vi "Edit.TestLauncher.vi"() -> ()   [LabVIEW 2019, in "Edit.lvclass"]
uses:
  Edit.lvclass
  <vilib>/JKI/JKI SMO/SMO/Typedefs/SMOState --Enum.ctl
  C:/Program Files (x86)/National Instruments/LabVIEW 2019/vi.lib/JKI/JKI SMO/SMO/SMO.lvclass
  <vilib>/JKI/JKI SMO/SMO/SMO.lvclass/SMO.ctl
  <vilib>/JKI/JKI SMO/SMO/Private/ReftoDVR--SMO.vi
  <vilib>/JKI/JKI SMO/SMO/SMO.lvclass
panel:
  out "SMO State":T1
  out "error out":errorcluster
  in  "Stop":bool
  # "Basic SMO Test Launcher"
  # "For instructions on how to use the JKI State Machine Objects, examples and video tutorials, visit:\nhttp://jki.net/state-machine-objects/\n\nJKI State Machine Objects™\nhttp://jki.net/state-machine-objects/\nCopyright (C) 2005-2015, JKI <info@jki.net>\nALL RIGHTS RESERVED"
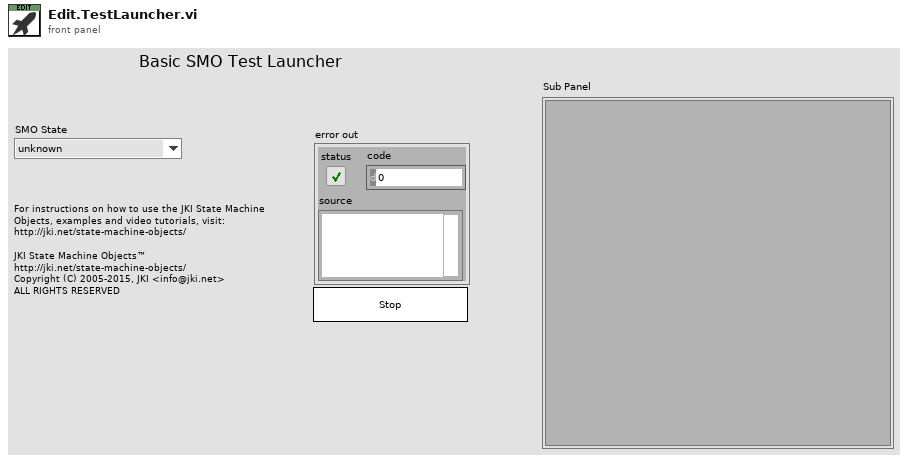
[diagram p1: front panel]
types:
  T1 = typedef "SMO.lvclass/SMOState --Enum.ctl" = enum16{"unknown", "Created", "Started", "Stopped"}
  T2 = typedef "SMO.lvclass/Public Events.ctl" = cluster{"Error":refnum<user-event>, "State":refnum<user-event>, "Reserve State":refnum<user-event>}
  T3 = cluster{"Event Registration Refnum":refnum<event-registration>}
  T4 = typedef "SMO.lvclass/RegisteredProcessData--Cluster.ctl" = cluster{"Name":string, "Static VI Ref":refnum<vi>, "Running":bool, "NotifierRef":u32}
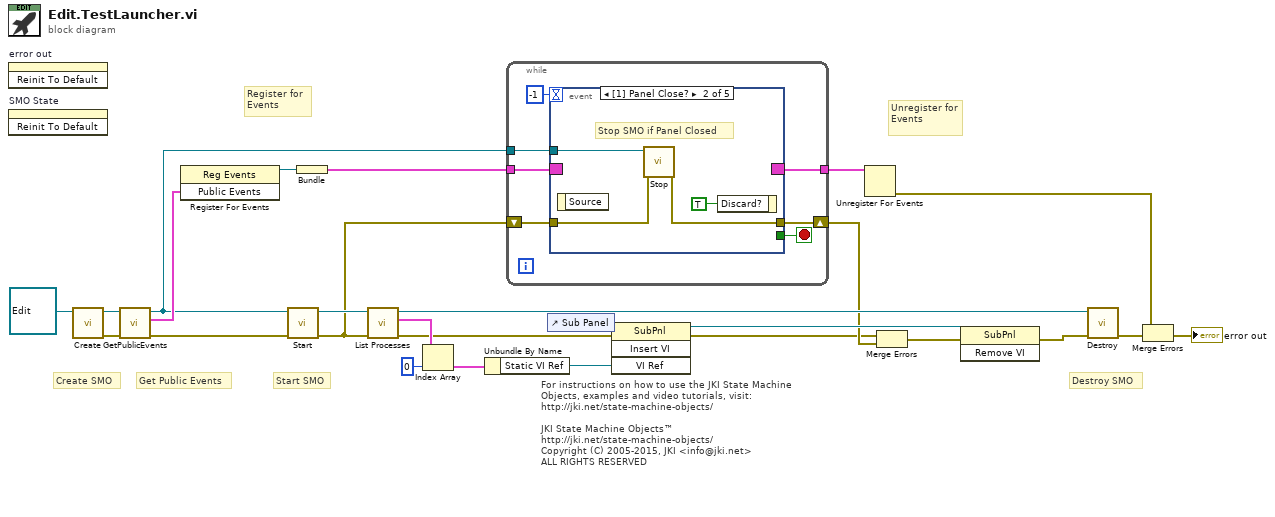
[diagram p0: block diagram]
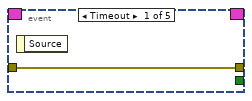
[diagram p2: hidden frame]
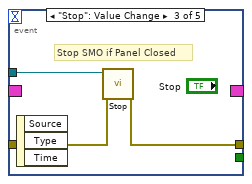
[diagram p3: hidden frame]
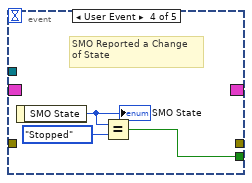
[diagram p4: hidden frame]
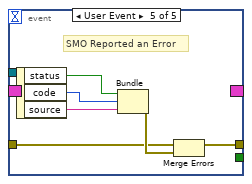
[diagram p5: hidden frame]
diagram:
  # "For instructions on how to use the JKI State Machine Objects, examples and video tutorials, visit:\nhttp://jki.net/state-machine-objects/\n\nJKI State Machine Objects™\nhttp://jki.net/state-machine-objects/\nCopyright (C) 2005-2015, JKI <info@jki.net>\nALL RIGHTS RESERVED"
  # "Get Public Events"
  # "Start SMO"
  # "Destroy SMO"
  # "Create SMO"
  # "Unregister for Events"
  # "Register for Events"
  n1 = invoke on="error out" class="Clust (strict)" method="Reinit To Default"() -> ()  [unwired: 3 in, 3 out]
  n2 = invoke on="SMO State" class="Enum (strict)" method="Reinit To Default"() -> ()  [unwired: 3 in, 3 out]
  n3 = call <vilib>:"Create.vi"("SMO"=refnum<class "Edit.lvclass"> refnum ("SMO.Template.lvclass")) -> ("error out"=w19:errorcluster, "SMO out"=w20:refnum<class "Edit.lvclass">)  [unwired: 8 in, 1 out]
  n4 = call <vilib>:"GetPublicEvents.vi"("error in (no error)"=w19, "SMO"=w20) -> ("error out"=w18:errorcluster, "Public Events"=w17:T2, "SMO out"=w12:refnum<class "Edit.lvclass">)  [unwired: 7 in]
  n5 = register-events(w17) -> (reference out=w16:refnum<event-registration>)  [unwired: 2 in, 1 out]
  n6 = call <vilib>:"Start.vi"("error in (no error)"=w18, "SMO"=w12) -> ("error out"=w5:errorcluster, "SMO out"=w7:refnum<class "Edit.lvclass">)  [unwired: 8 in]
  n7 = Bundle("Event Registration Refnum"=w16) -> (w25:T3)  [unwired: 1 in]
  n8 = call <vilib>:"List Processes.vi"("error in (no error)"=w5, "SMO"=w7) -> ("error out"=w1:errorcluster, "Registered Processes"=w4:T4[], "SMO out"=w6:refnum<class "Edit.lvclass">)  [unwired: 7 in]
  n9 = Index Array(array=w4, index=0) -> (element=w14:T4)
  n10 = Unbundle By Name(w14) -> ("Static VI Ref"=w13:refnum<vi>)
  n11 = while {
    shift-right: [w27] -> w3
    shift-left: w5 -> [w32]
    tunnel: w25 -> [w31]
    tunnel: [w30] -> w26
    tunnel: w12 -> [w29]
    stop <- w33 stop-if-true
    n12 = event shown="[1] Panel Close?" {
      selector: w31 -> [_ _ _ _ _]
      dyn-events: [_ _ _ _ _] -> w30
      timeout: -1 -> [_ _ _ _ _]
      tunnel: [_ _ _ w42 _] -> w33
      tunnel: w29 -> [_ w38 w41 _ _]
      tunnel: [w34 w37 w40 _ w48] -> w27
      tunnel: w32 -> [w34 w35 w39 _ w45]
      event Timeout {
        n13 = event-data() -> ()  [unwired: 1 in, 1 out]
      }
      event Panel Close? {
        # "Stop SMO if Panel Closed"
        n14 = event-data() -> ()  [unwired: 1 in, 1 out]
        n15 = call <vilib>:"Stop.vi"("error in (no error)"=w35, "SMO"=w38) -> ("error out"=w37:errorcluster)  [unwired: 8 in, 1 out]
        n16 = event-data("Discard?"=TRUE ("OK")) -> ()  [unwired: 1 in, 1 out]
      }
      event "Stop": Value Change {
        # "Stop SMO if Panel Closed"
        n17 = event-data() -> ()  [unwired: 1 in, 3 out]
        n18 = call <vilib>:"Stop.vi"("error in (no error)"=w39, "SMO"=w41) -> ("error out"=w40:errorcluster)  [unwired: 8 in, 1 out]
      }
      event User Event {
        # "SMO Reported a Change\nof State"
        n19 = event-data() -> ("SMO State"=w44:T1)  [unwired: 1 in]
        "SMO State" <- w44
        n20 = Equal?(x=w44, y=SMOState_--Enum."Stopped") -> (x = y?=w42:bool)
      }
      event User Event {
        # "SMO Reported an Error"
        n21 = event-data() -> ("status"=w47:bool, "code"=w50:i32, "source"=w49:string)  [unwired: 1 in]
        n22 = Bundle("status"=w47, "code"=w50, "source"=w49) -> (w46:errorcluster)  [unwired: 1 in]
        n23 = Merge Errors(w45, w46) -> (w48:errorcluster)
      }
    }
  }
  n24 = control-ref of="Sub Panel"() -> (w11:refnum<vi>)
  n25 = invoke class="SubPnl" method="Insert VI"(reference=w11, error in=w1, "VI Ref"=w13) -> (reference out=w8:refnum<vi>, error out=w2:errorcluster)  [unwired: 1 in, 2 out]
  n26 = Unregister For Events(event registration refnum=w26) -> (error out=w24:errorcluster)  [unwired: 1 in]
  n27 = Merge Errors(w2, w3) -> (w10:errorcluster)
  n28 = invoke class="SubPnl" method="Remove VI"(reference=w8, error in=w10) -> (error out=w9:errorcluster)  [unwired: 1 in, 2 out]
  n29 = call <vilib>:"Destroy.vi"("error in (no error)"=w9, "SMO"=w6) -> ("error out"=w22:errorcluster)  [unwired: 9 in]
  n30 = Merge Errors(w24, w22) -> (→"error out":errorcluster)
